vi "Cleanup (User).vi"(8 "error in":errorcluster, 11 "Node in":refnum<class "AMS Power Supply Template.lvclass">) -> (0 "error out":errorcluster caption="error in", 3 "Node out":refnum<class "AMS Power Supply Template.lvclass">)   [LabVIEW 2023, in "AMS Power Supply Template.lvlib" / "AMS Power Supply Template.lvclass"]
uses:
  AMS Power Supply Template.lvclass
  AMS Power Supply Template.lvclass/AMS Power Supply Template.ctl
  C:/Program Files/National Instruments/BLS plugin/Capabilities/Capabilities/High Level Capabilities/Power Supply/Output Enable Write Single.vi
  C:/Program Files/National Instruments/BLS plugin/Capabilities/Capabilities/High Level Capabilities/Power Supply/Power Supply.lvclass
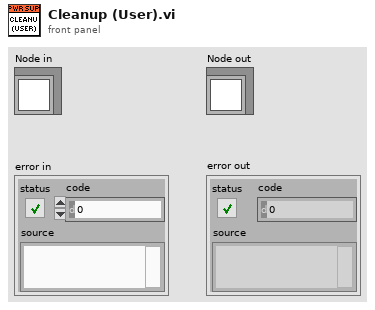
[diagram p1: front panel]
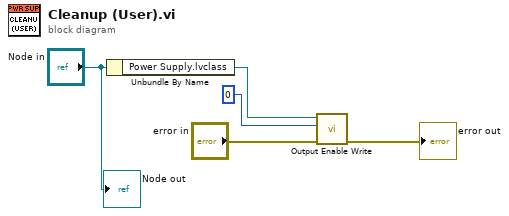
[diagram p0: block diagram]
diagram:
  n1 = Unbundle By Name("Node in") -> ("Power Supply.lvclass"=w2:refnum<class "Power Supply.lvclass">)
  n2 = call-poly "Output Enable Write.vi"("error in"="error in", "Output Enable STS"=0, "Power Supply In"=w2) -> ("error out"=→"error out":errorcluster)  [unwired: 7 in, 1 out]
  "Node out" <- "Node in"
